vi "AverageFilter.vi"(7 "Initialize":bool, 8 "Avg Len":i32, 11 "Input":dbl) -> (3 "Avg":dbl)   [LabVIEW 2010]
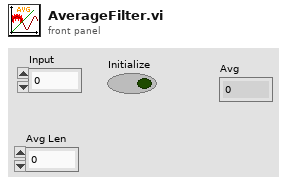
[diagram p1: front panel]
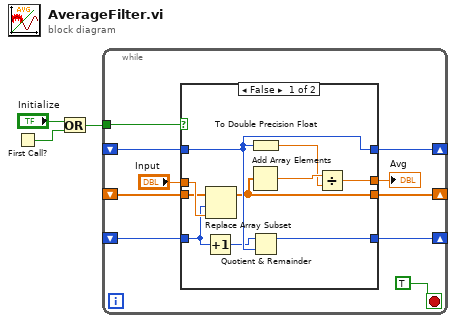
[diagram p0: block diagram]
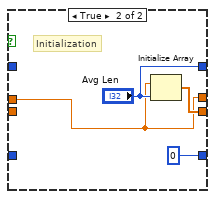
[diagram p2: hidden frame]
diagram:
  n1 = First Call?() -> (First Call?: T/F=w2:bool)
  n2 = Or(x="Initialize", y=w2) -> (x .or. y?=w3:bool)
  n3 = while {
    tunnel: w3 -> [w12]
    shift-right: [w11] -> _
    shift-left: _ -> [w8]
    shift-right: [w10] -> _
    shift-left: _ -> [w7]
    shift-right: [w9] -> _
    shift-left: _ -> [w6]
    stop <- TRUE stop-if-true
    n4 = case shown="False" w12 {
      tunnel: [w17 w25] -> w11
      tunnel: [w21 "Avg Len"] -> w10
      tunnel: [w15 0 ("index")] -> w9
      tunnel: w8 -> [w18 _]
      tunnel: w7 -> [w21 _]
      tunnel: w6 -> [w14 _]
      tunnel: "Input" -> [w20 w24]
      tunnel: [w16 w24] -> w4
      frame False {
        n5 = Increment(x=w14) -> (x+1=w19:i32)
        n6 = Replace Array Subset(array=w18, new element=w20, index=w14) -> (w17:dbl[])
        n7 = Add Array Elements(numeric array=w17) -> (sum=w23:dbl)
        n8 = To Double Precision Float(number=w21) -> (double precision float=w22:dbl)
        n9 = Quotient & Remainder(x=w19, y=w21) -> (x-y*floor(x/y)=w15:i32)  [unwired: 1 out]
        n10 = Divide(x=w23, y=w22) -> (x/y=w16:dbl)
      }
      frame True {
        # "Initialization"
        n11 = Initialize Array(w24, "Avg Len") -> (w25:dbl[])
      }
    }
    "Avg" <- w4
  }
